vi "KE622x -- 2182 -A Get Range.vi"(0 "622x Resource In":refnum<visa-resource-name>, 1 "Check For SCPI Errors? (T)":bool=TRUE, 11 "error in (no error)":errorcluster) -> (4 "622x Resource Out (dupl)":refnum<visa-resource-name>, 8 "2182/2182A Range":enum16{"10mV", "100mV", "1V", "10V", "100V"}(ring), 15 "error out":errorcluster)   [LabVIEW 2013, in "Keithly user program.lvlib"]
uses:
  Keithly user program.lvlib
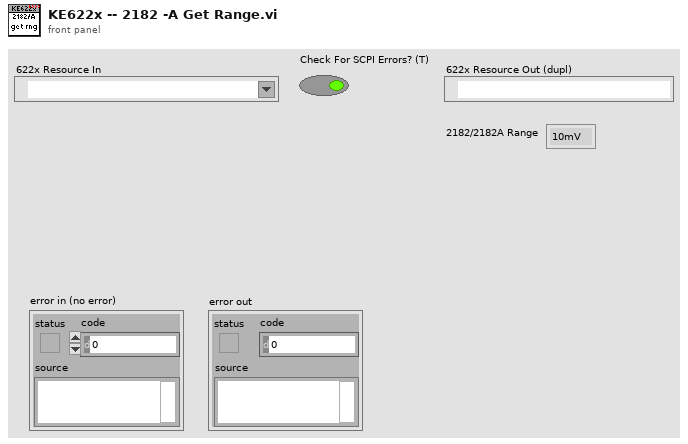
[diagram p1: front panel]
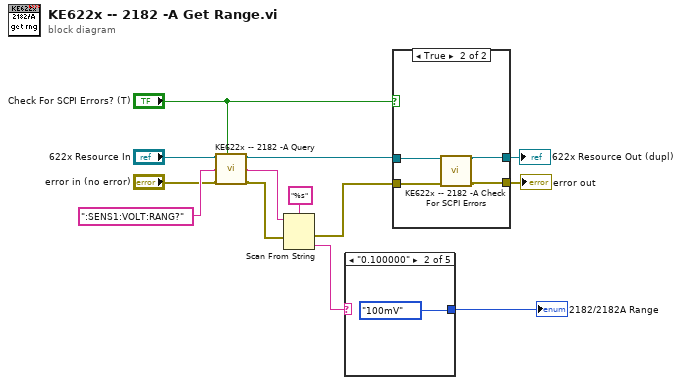
[diagram p0: block diagram]
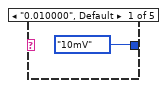
[diagram p2: hidden frame]
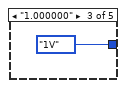
[diagram p3: hidden frame]
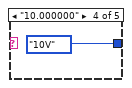
[diagram p4: hidden frame]
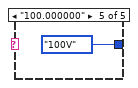
[diagram p5: hidden frame]
diagram:
  n1 = call "KE622x -- 2182 -A Query.vi"("622x Resource In"="622x Resource In", "Check For SCPI Errors? (T)"="Check For SCPI Errors? (T)", "2182-A Write String"=":SENS1:VOLT:RANG?", "error in (no error)"="error in (no error)") -> ("622x Resource Out (dupl)"=w3:refnum<visa-resource-name>, "2182-A Reponse String"=w7:string, "error out"=w5:errorcluster)  [unwired: 9 in]
  n2 = Scan From String(format string="%s", input string=w7, error in=w5) -> (error out=w12:errorcluster, output 1=w9:string)  [unwired: 2 in, 2 out]
  n3 = case shown="\"0.100000\"" w9 {
    tunnel: [enum16{"10mV", "100mV", "1V", "10V", "100V"}."10mV" ("2182/2182A Range") enum16{"10mV", "100mV", "1V", "10V", "100V"}."100mV" ("2182/2182A Range") enum16{"10mV", "100mV", "1V", "10V", "100V"}."1V" ("2182/2182A Range") enum16{"10mV", "100mV", "1V", "10V", "100V"}."10V" ("2182/2182A Range") enum16{"10mV", "100mV", "1V", "10V", "100V"}."100V" ("2182/2182A Range")] -> w1
    frame "0.010000", Default {
    }
    frame "0.100000" {
    }
    frame "1.000000" {
    }
    frame "10.000000" {
    }
    frame "100.000000" {
    }
  }
  "2182/2182A Range" <- w1
  n4 = case shown="True" "Check For SCPI Errors? (T)" {
    tunnel: w3 -> [w20 w24]
    tunnel: w12 -> [w19 w22]
    tunnel: [w20 w23] -> w11
    tunnel: [w19 w21] -> w10
    frame False {
    }
    frame True {
      n5 = call "KE622x -- 2182 -A Check For SCPI Errors.vi"("VISA Resource In"=w24, "error in (no error)"=w22) -> ("VISA Resource Out (dupl)"=w23:refnum<visa-resource-name>, "error out"=w21:errorcluster)  [unwired: 10 in, 2 out]
    }
  }
  "622x Resource Out (dupl)" <- w11
  "error out" <- w10
